vi "open_sysconfig_session.vi"(8 "error in (no error)":errorcluster, 10 "Target Access":T1, 11 "DevInfo":T2={"Hostname"="", "IPAddress"="", "MAC"="", "SerialNum"="", "Model"="", "Status"="", "FW"="", "OSDesc"="", "ImgTitle"="", "ImgDesc"="", "ImgVer"="", "ImgID"="", "IP Address Request Mode"=1, "SubnetMask"="", "Gateway"="", "DNSServer"=""} {"IP Address Request Mode" items=["Static"=1, "DHCP/Link-Local"=2, "Link-Local Only"=4, "DHCP Only"=8]}) -> (0 "error out":errorcluster, 2 "Cancelled":bool, 3 "Session Out":refnum<k21>)   [LabVIEW 2021]
uses:
  TypeDefs/DevInfo.ctl
  TypeDefs/TargetAccess.ctl
  <vilib>/nisyscfg/Close (System).vi
  <vilib>/nisyscfg/nisyscfg.lvlib
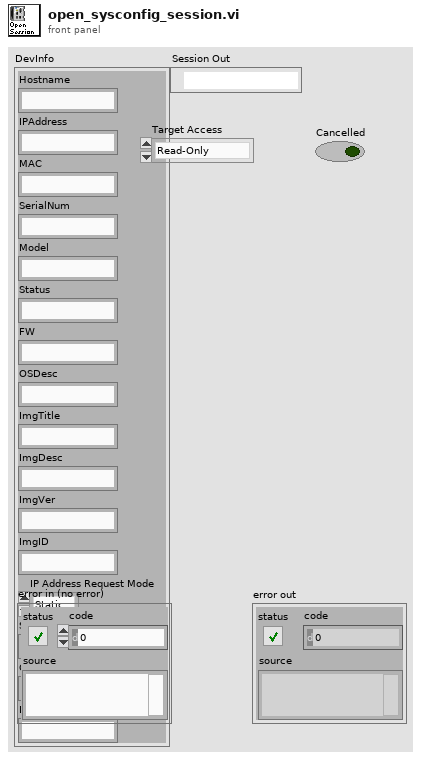
[diagram p1: front panel]
types:
  T1 = typedef "TargetAccess.ctl" = enum16{"Read-Only", "Admin"}
  T2 = typedef "DevInfo.ctl" = cluster{"Hostname":string, "IPAddress":string, "MAC":string, "SerialNum":string, "Model":string, "Status":string, "FW":string, "OSDesc":string, "ImgTitle":string, "ImgDesc":string, "ImgVer":string, "ImgID":string, "IP Address Request Mode":i32, "SubnetMask":string, "Gateway":string, "DNSServer":string}
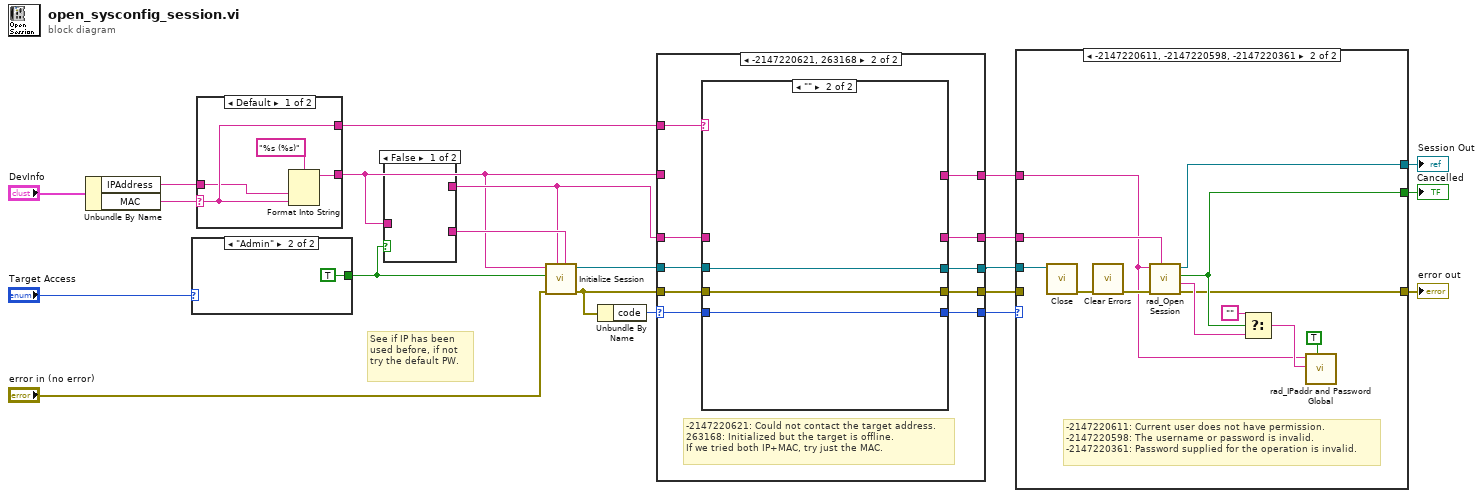
[diagram p0: block diagram]
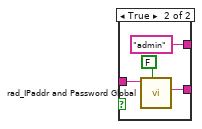
[diagram p2: hidden frame]
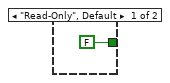
[diagram p3: hidden frame]
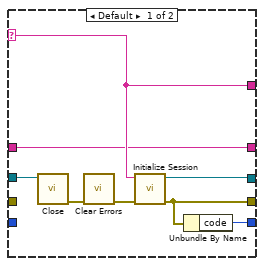
[diagram p7: hidden frame]
diagram:
  # "See if IP has been used before, if not try the default PW."
  n1 = Unbundle By Name("DevInfo") -> ("IPAddress"=w11:string, "MAC"=w10:string)
  n2 = case shown="\"Admin\"" "Target Access" {
    tunnel: [FALSE TRUE] -> w2
    frame "Read-Only", Default {
    }
    frame "Admin" {
    }
  }
  n3 = case shown="Default" w10 {
    selector: w10 -> [w25 _]
    tunnel: [w26 w28] -> w3
    tunnel: [w25 _] -> w12
    tunnel: w11 -> [w24 w28]
    frame Default {
      n4 = Format Into String(format string="%s (%s)", w24, w25) -> (resulting string=w26:string)  [unwired: 2 in, 1 out]
    }
    frame "" {
    }
  }
  n5 = case shown="False" w2 {
    tunnel: w3 -> [_ w32]
    tunnel: [_ w31] -> w13
    tunnel: [_ "admin" ("User Name")] -> w4
    frame False {
    }
    frame True {
      n6 = call "rad_IPaddr and Password Global.vi"("Read(F)/Write(T)"=FALSE, "IP/MAC Address"=w32) -> ("Password"=w31:string)  [unwired: 8 in, 1 out]
    }
  }
  n7 = call <vilib>:"Initialize Session.vi"("Password"=w13, "User Name"=w4, "error in (no error)"="error in (no error)", "Force Property Refresh (T)"=w2, "Target (localhost)"=w3) -> ("error out"=w9:errorcluster, "Session out"=w8:refnum<k21>)  [unwired: 5 in]
  n8 = Unbundle By Name(w9) -> ("code"=w7:i32)
  n9 = case shown="-2147220621, 263168" w7 {
    selector: w7 -> [w35 w41]
    tunnel: w8 -> [w37 w45]
    tunnel: w9 -> [w36 w46]
    tunnel: w12 -> [_ w47]
    tunnel: [w36 w44] -> w16
    tunnel: [w35 w43] -> w14
    tunnel: [w37 w42] -> w15
    tunnel: w3 -> [w34 _]
    tunnel: [w34 w40] -> w17
    tunnel: [w33 w39] -> w18
    tunnel: w4 -> [w33 w38]
    frame Default {
    }
    frame -2147220621, 263168 {
      # "-2147220621: Could not contact the target address.\n263168: Initialized but the target is offline.\nIf we tried both IP+MAC, try just the MAC."
      n10 = case shown="\"\"" w47 {
        selector: w47 -> [w49 _]
        tunnel: w46 -> [_ w57]
        tunnel: w45 -> [w53 w58]
        tunnel: [w52 w57] -> w44
        tunnel: [w51 w56] -> w43
        tunnel: [w50 w58] -> w42
        tunnel: w41 -> [_ w56]
        tunnel: [w49 _] -> w40
        tunnel: [w48 _] -> w39
        tunnel: w38 -> [w48 _]
        frame Default {
          n11 = call-poly <vilib>:"Close.vi"("Session in"=w53) -> ("error out"=w55:errorcluster)  [unwired: 10 in]
          n12 = call <vilib>:"Clear Errors.vi"("error in (no error)"=w55) -> ("error out"=w54:errorcluster)  [unwired: 5 in, 1 out]
          n13 = call <vilib>:"Initialize Session.vi"("error in (no error)"=w54, "Target (localhost)"=w49) -> ("error out"=w52:errorcluster, "Session out"=w50:refnum<k21>)  [unwired: 8 in]
          n14 = Unbundle By Name(w52) -> ("code"=w51:i32)
        }
        frame "" {
        }
      }
    }
  }
  n15 = case shown="-2147220611, -2147220598, -2147220361" w14 {
    tunnel: [w60 w67] -> w19
    tunnel: w15 -> [w60 w72]
    tunnel: w16 -> [w59 _]
    tunnel: w17 -> [_ w62]
    tunnel: w18 -> [_ w68]
    tunnel: [w59 w61] -> w20
    tunnel: [_ w65] -> w21
    frame Default {
    }
    frame -2147220611, -2147220598, -2147220361 {
      # "-2147220611: Current user does not have permission.\n-2147220598: The username or password is invalid.\n-2147220361: Password supplied for the operation is invalid."
      n16 = call-poly <vilib>:"Close.vi"("Session in"=w72) -> ("error out"=w71:errorcluster)  [unwired: 10 in]
      n17 = call <vilib>:"Clear Errors.vi"("error in (no error)"=w71) -> ("error out"=w69:errorcluster)  [unwired: 5 in, 1 out]
      n18 = call "rad_Open Session.vi"("User name"=w68, "error in (no error)"=w69, "Target Address"=w62) -> ("error out"=w61:errorcluster, "Password Out"=w64:string, "Cancelled"=w65:bool, "session out"=w67:refnum<k21>)  [unwired: 5 in]
      n19 = Select(t="", s=w65, f=w64) -> (s? t:f=w63:string)
      n20 = call "rad_IPaddr and Password Global.vi"("Read(F)/Write(T)"=TRUE, "Password"=w63, "IP/MAC Address"=w62) -> ()  [unwired: 7 in, 2 out]
    }
  }
  "Cancelled" <- w21
  "error out" <- w20
  "Session Out" <- w19
